vi "create_from_json.vi"(8 "error in":errorcluster, 11 "JSON":string) -> (0 "error out":errorcluster, 2 "Workspace":refnum<class "workspace.lvclass">)   [LabVIEW 2020, in "nominal types.lvlib" / "workspace.lvclass"]
uses:
  workspace.lvclass
  workspace.lvclass/workspace.ctl
  aec5e6cc-91bd-4b97-98ba-b813f6ae0012.vi
  <vilib>/JDP Science/JSONtext/Find Item.vi
  <vilib>/JDP Science/JSONtext/Next JSON Value.vi
  <vilib>/JDP Science/JSONtext/String Subset.vi
  <vilib>/JDP Science/JSONtext/Parsing/Advance past next JSON Value (inlined COPY).vi
  <vilib>/JDP Science/JSONtext/Parsing/Advance past whitespace.vi
  <vilib>/JDP Science/JSONtext/Parsing/Advance past String.vi
  <vilib>/JDP Science/JSONtext/Parsing/Advance past Number.vi
  <vilib>/JDP Science/JSONtext/Parsing/Advance past Line Ending.vi
  <vilib>/JDP Science/JSONtext/Parsing/Parse Full Path or Item Name.vi
  <vilib>/JDP Science/JSONtext/Parsing/Advance past Array.vi
  <vilib>/JDP Science/JSONtext/Parsing/Advance past Object.vi
  <vilib>/JDP Science/JSONtext/support/Error Cluster From Code.vi
  <vilib>/JDP Science/JSONtext/Offset/Find Item Locations by Path.vi
  <vilib>/JDP Science/JSONtext/JSON text to Variant.vi
  <vilib>/JDP Science/JSONtext/LVClass Serializer/JSONtext LVClass Serializer.lvclass
  <vilib>/JDP Science/JSONtext/JSONtext.lvlib
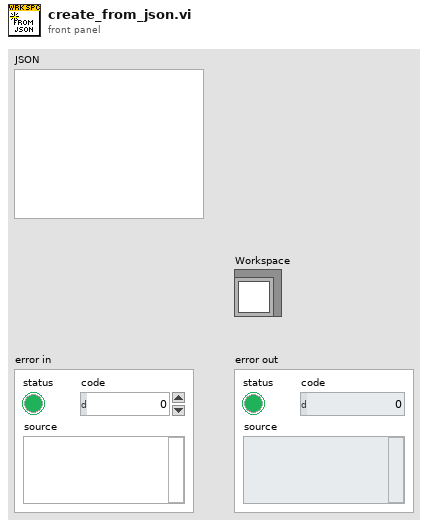
[diagram p1: front panel]
types:
  T1 = cluster{"[0]":string, "[1]":string, "[2]":string, "[3]":string}
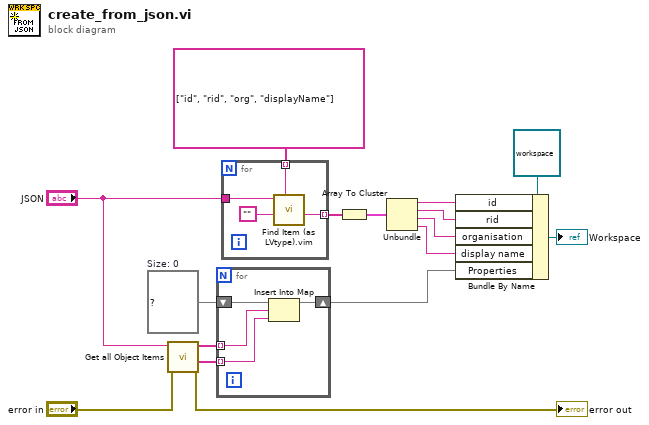
[diagram p0: block diagram]
diagram:
  w16 = map{string, string} {}  # Size: 0
  n1 = call <vilib>:"Get all Object Items.vi"("error in (no error)"="error in", "JSON"="JSON") -> ("error out"=→"error out":errorcluster, "<JSON>"=w14:string[], "Item Names"=w15:string[])  [unwired: 6 in, 1 out]
  n2 = for {
    shift-right: [w17] -> w3
    shift-left: w16 -> [w20]
    tunnel: w15 -> [w19] mode=indexing
    tunnel: w14 -> [w18] mode=indexing
    n3 = Insert Into Map(map in=w20, key=w19, value=w18) -> (map out=w17:map{string, string})  [unwired: 2 out]
  }
  n4 = for {
    tunnel: string[] ["id", "rid", "org", "displayName"] ("$Path or Item Name") -> [w23] mode=indexing
    tunnel: "JSON" -> [w22]
    tunnel: [w21] -> w10 mode=indexing
    n5 = call "Find Item (as LVtype).vim"("$Path or Item Name"=w23, "Data Type and Default Value"="", "JSON"=w22) -> ("Data"=w21:string)  [unwired: 5 in, 3 out]
  }
  n6 = Array To Cluster(array=w10) -> (cluster=w9:T1)
  n7 = Unbundle(w9) -> ("[0]"=w8:string, "[1]"=w7:string, "[2]"=w6:string, "[3]"=w5:string)
  n8 = Bundle By Name(cluster=refnum<class "workspace.lvclass"> refnum ("Workspace"), "id"=w8, "rid"=w7, "organisation"=w6, "display name"=w5, "Properties"=w3) -> (→"Workspace":refnum<class "workspace.lvclass">)
